vi "Day 1 Puzzle 1.vi"(11 "Path":path) -> (3 "Snacks sum list":i64[](array[numeric]))   [LabVIEW 2021]
uses:
  <vilib>/Utility/file.llb/Read Delimited Spreadsheet (I64).vi
panel:
  out "max value":i64
  out "subarray":i64[](array[numeric])
  out "error out":errorcluster
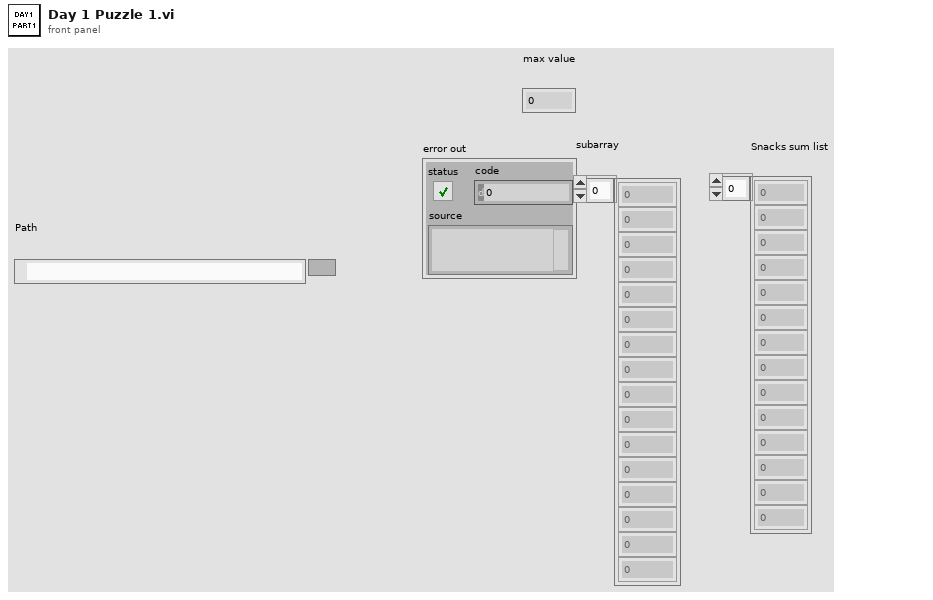
[diagram p1: front panel]
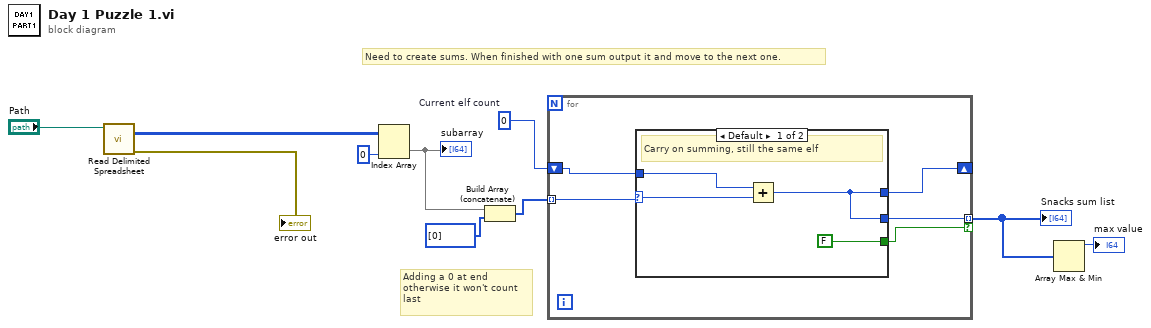
[diagram p0: block diagram]
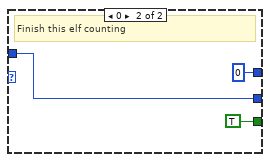
[diagram p2: hidden frame]
diagram:
  w6 = i64 0  # Current elf count
  # "Adding a 0 at end\notherwise it won't count\nlast"
  # "Need to create sums. When finished with one sum output it and move to the next one."
  n1 = call-poly <vilib>:"Read Delimited Spreadsheet.vi"("file path (dialog if empty)"="Path") -> ("all rows"=w8:i64[][], "error out"=→"error out":errorcluster)  [unwired: 9 in, 4 out]
  n2 = Index Array(array=w8, index (col)=0 ("disabled index (col)")) -> (element=w5:i64[])  [unwired: 1 in]
  "subarray" <- w5
  n3 = Build Array (concatenate)(w5, i64[] [0] ("array")) -> (w3:i64[])
  n4 = for {
    tunnel: w3 -> [w15] mode=indexing
    shift-right: [w13] -> _
    shift-left: w6 -> [w14]
    tunnel: [w12] -> w2 mode=indexing if=w11
    n5 = case shown="Default" w15 {
      selector: w15 -> [w18 _]
      tunnel: w14 -> [w19 w21]
      tunnel: [w17 i64 0] -> w13
      tunnel: [w17 w21] -> w12
      tunnel: [FALSE TRUE] -> w11
      frame Default {
        # "Carry on summing, still the same elf"
        n6 = Add(x=w19, y=w18) -> (x+y=w17:i64)
      }
      frame 0 {
        # "Finish this elf counting"
      }
    }
  }
  "Snacks sum list" <- w2
  n7 = Array Max & Min(array=w2) -> (max value=→"max value":i64)  [unwired: 3 out]
